vi "lab4_5.vi"() -> ()   [LabVIEW 2021]
panel:
  out "Numeric":i32
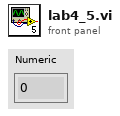
[diagram p1: front panel]
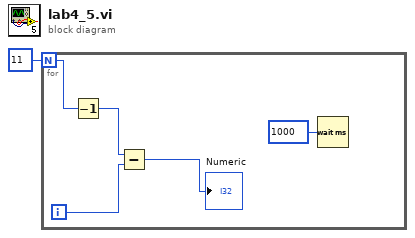
[diagram p0: block diagram]
diagram:
  n1 = for {
    N: 11 -> [w6]
    i -> [w4]
    n2 = Decrement(x=w6) -> (x-1=w5:i32)
    n3 = Subtract(x=w5, y=w4) -> (x-y=→"Numeric":i32)
    n4 = Wait (ms)(milliseconds to wait=u32 1000) -> ()  [unwired: 1 out]
  }
